vi "push_raster_data_as_CS.vi"(6 "number-of-pixels":i32=512, 8 "error in":errorcluster, 10 "fpga_input_vec":dbl[](array[numeric]), 11 "FPGA Interface":T1) -> (0 "error out":errorcluster, 3 "FPGA Interface out":T1)   [LabVIEW 2017]
uses:
  fpga_interface_lib/fpga_interface_types/HOST_to_FPGA_FXP_16-5_FIFO_interface.ctl
  <vilib>/Utility/error.llb/Error Cluster From Error Code.vi
  <vilib>/rvi/errors/niLvFpgaAdjustHostInterfaceError.vi
  <vilib>/rvi/interface/nirviMethod/nirviMethod.xnode
  fpga_interface_lib/fpga_interface.lvlib
  <vilib>/FPGAPlugInAG/Dynamic/niLvFpga_WriteFifo_Dynamic.vi
  <vilib>/rvi/errors/niLvFpgaMergeErrorWithErrorCode.vi
panel:
  out "Numeric":i32
  out "meta idx":dbl[](graph)
  out "base x_ref":dbl[](graph)
  out "base y_ref":dbl[](graph)
  out "elements left":i32=1
  # "Debug only! (disabled in block diagram)"
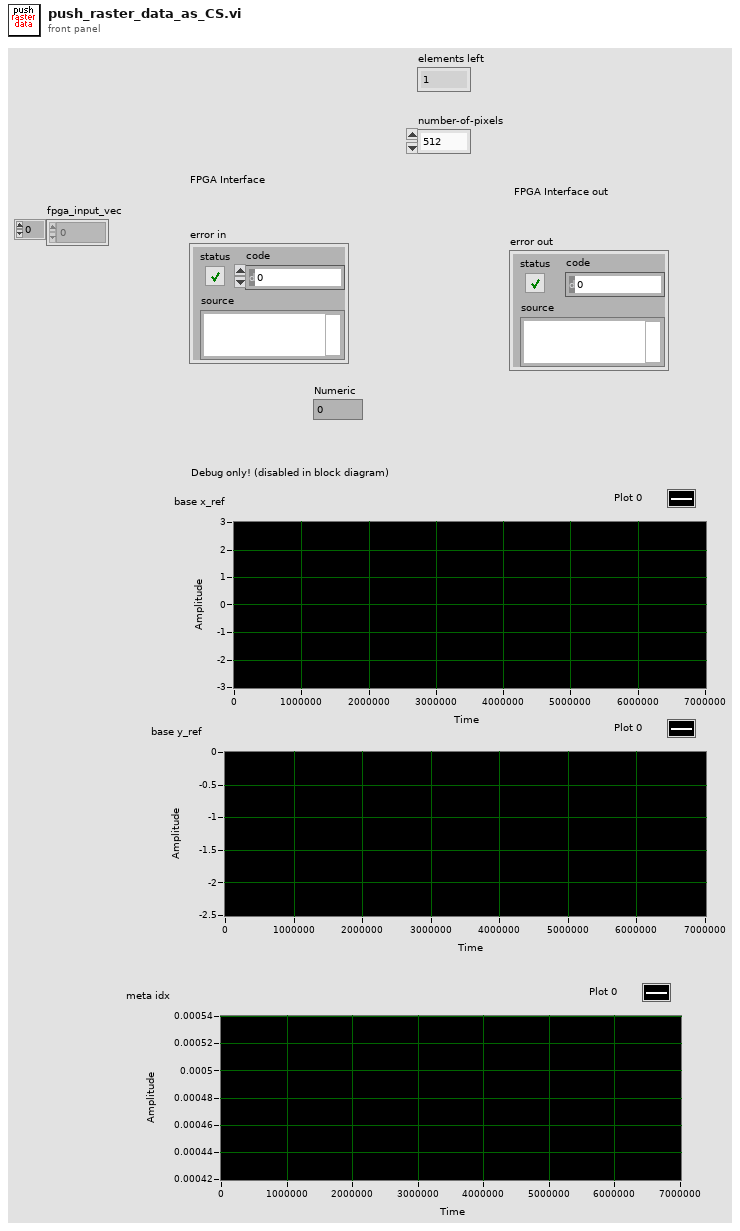
[diagram p1: front panel]
types:
  T1 = typedef "fpga_interface.lvlib/HOST_to_FPGA_FXP_16-5_FIFO_interface.ctl" = refnum<k20>
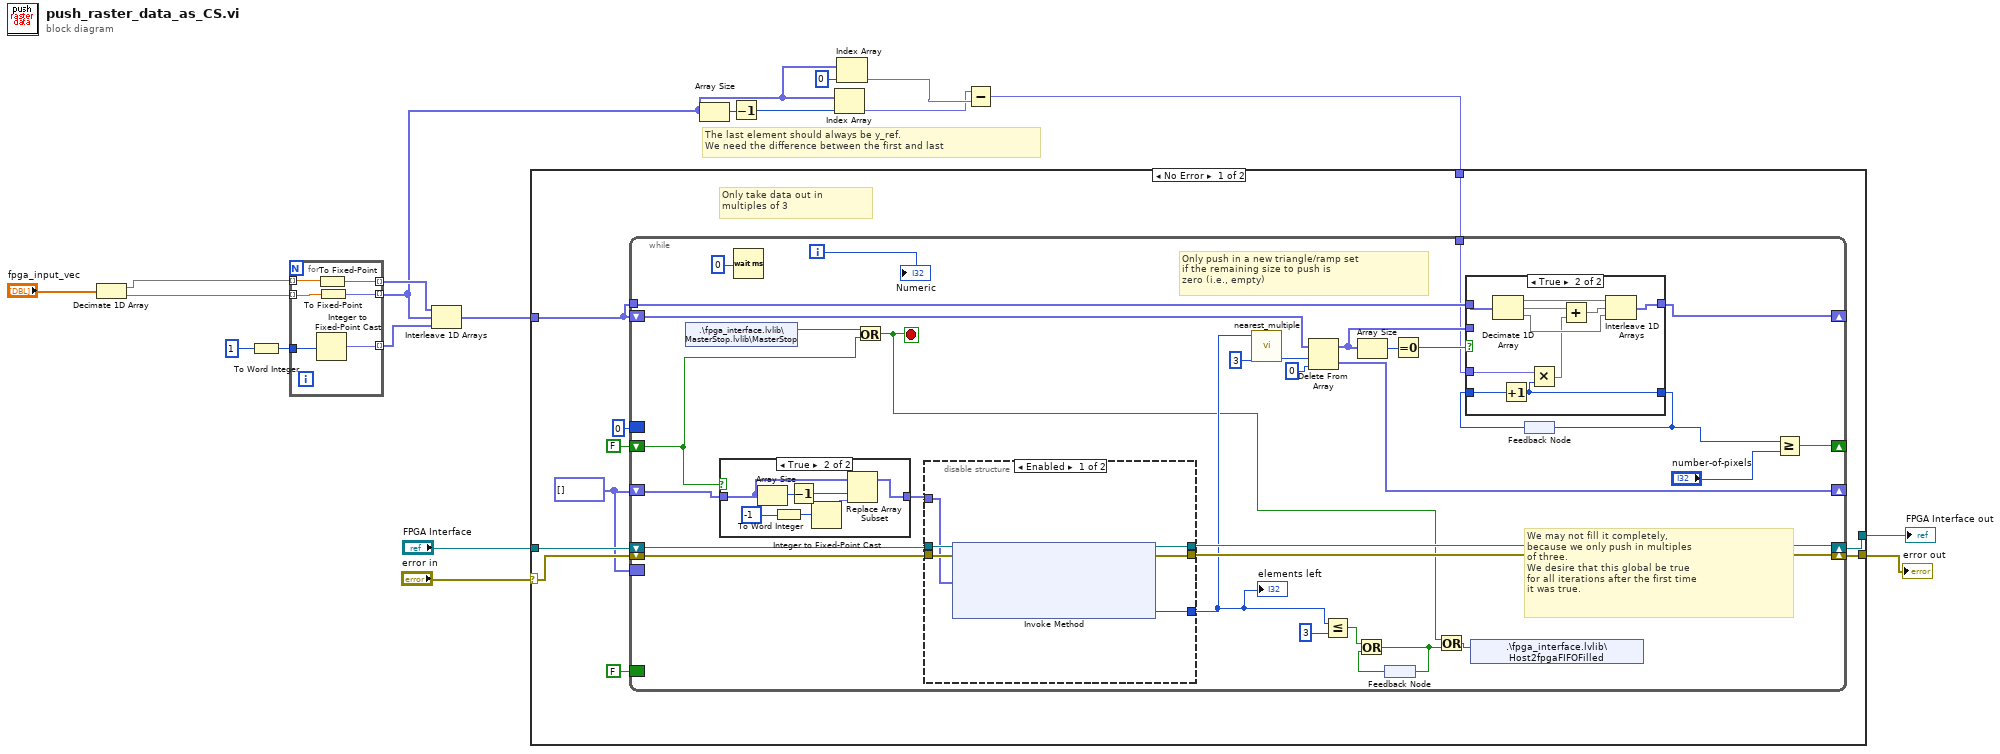
[diagram p0: block diagram]
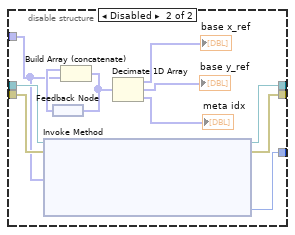
[diagram p4: hidden frame]
diagram:
  # "The last element should always be y_ref.\nWe need the difference between the first and last"
  n1 = Decimate 1D Array("fpga_input_vec") -> (w8:dbl[], w7:dbl[])
  n2 = To Word Integer(number=i16 1) -> (16bit integer=w18:i16)
  n3 = for {
    tunnel: w8 -> [w25] mode=indexing
    tunnel: w7 -> [w24] mode=indexing
    tunnel: [w23] -> w5 mode=indexing
    tunnel: [w22] -> w17 mode=indexing
    tunnel: w18 -> [w21]
    tunnel: [w20] -> w12 mode=indexing
    n4 = Integer to Fixed-Point Cast(integer=w21) -> (fixed-point=w20:fxp<+/-,16,5>)  [unwired: 1 in]
    n5 = To Fixed-Point(number=w25) -> (fixed-point=w22:fxp<+/-,16,5>)  [unwired: 1 in]
    n6 = To Fixed-Point(number=w24) -> (fixed-point=w23:fxp<+/-,16,5>)  [unwired: 1 in]
  }
  n7 = Interleave 1D Arrays(w17, w5, w12) -> (w13:fxp<+/-,16,5>[])
  n8 = Array Size(array=w5) -> (size(s)=w10:i32)
  n9 = Decrement(x=w10) -> (x-1=w9:i32)
  n10 = Index Array(array=w5, index=w9) -> (element=w2:fxp<+/-,16,5>)
  n11 = Index Array(array=w5, index=0) -> (element=w3:fxp<+/-,16,5>)
  n12 = Subtract(x=w2, y=w3) -> (x-y=w1:fxp<+/-,17,6>)
  n13 = case shown="No Error" "error in" {
    selector: "error in" -> [w29 w105]
    tunnel: "FPGA Interface" -> [w34 w106]
    tunnel: [w33 w105] -> w15
    tunnel: [w32 w106] -> w14
    tunnel: w13 -> [w30 _]
    tunnel: w1 -> [w28 _]
    frame No Error {
      w27 = fxp<+/-,16,5>[] []
      # "Only take data out in \nmultiples of 3"
      n14 = while {
        shift-right: [w49] -> _
        shift-left: w30 -> [w67]
        border: 0 ("Timeout (ms)") -> [_]
        shift-right: [w51] -> w33
        shift-left: w29 -> [w54]
        shift-right: [w52] -> w32
        shift-left: w34 -> [w55]
        shift-right: [w58] -> _
        shift-left: FALSE -> [w46]
        border: w27 -> [_]
        tunnel: w30 -> [w56]
        shift-right: [w53] -> _
        shift-left: w27 -> [w47]
        tunnel: w28 -> [w44]
        border: FALSE -> [_]
        i -> [w36]
        stop <- w37 stop-if-true
        # "We may not fill it completely,\nbecause we only push in multiples\nof three. \nWe desire that this global be true\nfor all iterations after the first time\nit was true."
        # "Only push in a new triangle/ramp set\nif the remaining size to push is\nzero (i.e., empty)"
        n15 = shared-variable ".\\fpga_interface.lvlib\\MasterStop.lvlib\\MasterStop"() -> (w60:bool)  [unwired: 1 in, 1 out]
        n16 = case shown="True" w46 {
          tunnel: [w68 w75] -> w48
          tunnel: w47 -> [w68 w69]
          frame False {
          }
          frame True {
            n17 = Array Size(array=w69) -> (size(s)=w74:i32)
            n18 = To Word Integer(number=i16 -1) -> (16bit integer=w70:i16)
            n19 = Decrement(x=w74) -> (x-1=w73:i32)
            n20 = Integer to Fixed-Point Cast(integer=w70) -> (fixed-point=w71:fxp<+/-,16,5>)  [unwired: 1 in]
            n21 = Replace Array Subset(array=w69, new element=w71, index=w73) -> (w75:fxp<+/-,16,5>[])
          }
        }
        n22 = Wait (ms)(milliseconds to wait=0) -> ()  [unwired: 1 out]
        n23 = Or(x=w60, y=w46) -> (x .or. y?=w37:bool)
        n24 = disable-structure shown="Enabled" {
          disable-tunnel: [w93 w96] -> w43
          disable-tunnel: [w92 w94] -> w51
          disable-tunnel: w55 -> [w91 w99]
          disable-tunnel: w54 -> [w90 w98]
          disable-tunnel: [w89 w95] -> w52
          disable-tunnel: w48 -> [w88 w97]
          frame Enabled {
            n25 = xnode "Invoke Method"("FPGA VI Reference In"=w91, "error in"=w90, "Data"=w88) -> ("FPGA VI Reference Out"=w89:T1, "error out"=w92:errorcluster, "Empty Elements Remaining"=w93:u32)  [unwired: 1 in]
          }
          frame Disabled {
            n26 = xnode "Invoke Method"("FPGA VI Reference In"=w99, "error in"=w98, "Data"=w97) -> ("FPGA VI Reference Out"=w95:T1, "error out"=w94:errorcluster, "Empty Elements Remaining"=w96:u32)  [unwired: 1 in]
            n27 = feedback #1() -> (w103:fxp<+/-,16,5>[])
            n28 = Build Array (concatenate)(w103, w97) -> (w104:fxp<+/-,16,5>[])
            n29 = feedback-in #1(w104) -> ()
            n30 = Decimate 1D Array(w104) -> (→"base x_ref":fxp<+/-,16,5>[], →"base y_ref":fxp<+/-,16,5>[], →"meta idx":fxp<+/-,16,5>[])
          }
        }
        "elements left" <- w43
        n31 = call "nearest_multiple.vi"("numChan"=u32 3 ("Empty Elements Remaining"), "N"=w43) -> ("(int) y*floor(x/y)"=w65:u64)  [unwired: 9 in]
        n32 = Delete From Array(array=w67, length=w65, index=0) -> (deleted portion=w53:fxp<+/-,16,5>[], array with subset deleted=w63:fxp<+/-,16,5>[])
        n33 = Less Or Equal?(x=w43, y=u32 3) -> (x <= y?=w41:bool)
        n34 = Array Size(array=w63) -> (size(s)=w50:i32)
        n35 = feedback #2() -> (w40:bool)
        n36 = Or(x=w41, y=w40) -> (x .or. y?=w39:bool)
        n37 = feedback-in #2(w39) -> ()
        n38 = Equal To 0?(x=w50) -> (x = 0?=w45:bool)
        n39 = Or(x=w37, y=w39) -> (x .or. y?=w38:bool)
        n40 = shared-variable ".\\fpga_interface.lvlib\\Host2fpgaFIFOFilled"(w38) -> ()  [unwired: 1 in, 1 out]
        n41 = feedback #3() -> (w61:i32)
        n42 = case shown="True" w45 {
          tunnel: [w77 w85] -> w49
          tunnel: w63 -> [w77 _]
          tunnel: w56 -> [_ w87]
          tunnel: w44 -> [_ w79]
          tunnel: [w76 w80] -> w59
          tunnel: w61 -> [w76 w84]
          frame False {
          }
          frame True {
            n43 = Decimate 1D Array(w87) -> (w86:fxp<+/-,16,5>[], w82:fxp<+/-,16,5>[], w81:fxp<+/-,16,5>[])
            n44 = Increment(x=w84) -> (x+1=w80:i32)
            n45 = Multiply(x=w79, y=w80) -> (x*y=w78:fxp<+/-,48,37>)
            n46 = Add(x=w82, y=w78) -> (x+y=w83:fxp<+/-,16,5>[])
            n47 = Interleave 1D Arrays(w86, w83, w81) -> (w85:fxp<+/-,16,5>[])
          }
        }
        n48 = feedback-in #3(w59) -> ()
        n49 = Greater Or Equal?(x=w59, y="number-of-pixels") -> (x >= y?=w58:bool)
        "Numeric" <- w36
      }
    }
    frame Error {
    }
  }
  "error out" <- w15
  "FPGA Interface out" <- w14
